vi "First_VI.vi"() -> ()   [LabVIEW 2011]
panel:
  out "Slide 2":dbl(slide) scale=0.0..10.0
  in  "Slide":dbl(slide) scale=0.0..10.0
  in  "Input":bool
  out "Output":bool
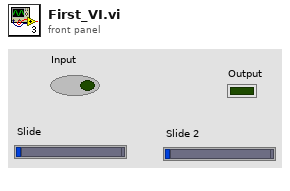
[diagram p1: front panel]
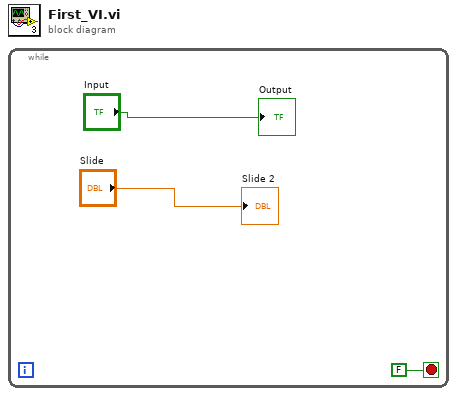
[diagram p0: block diagram]
diagram:
  n1 = while {
    stop <- FALSE stop-if-true
    "Output" <- "Input"
    "Slide 2" <- "Slide"
  }
